vi "Jog_Home_Device_Travel_Range.vi"() -> ()   [LabVIEW 2017]
uses:
  U:/UDocuments/Thorlabs.Elliptec.ELLO_DLL.dll
  Thorlabs.Elliptec.ELLO_DLL.dll
panel:
  out "Stage Position (mm/degrees)":dbl
  out "?":string[](array[string])
  in  "Jog Step Size (mm/degrees)":dbl
  in  "Homing Direction":i32(ring)=48 items=["Linear, Clockwise"=48, "AntiClockwise"=49]
  in  "Device Address":string
  in  "?":bool
  in  "?":bool
  in  "Stop VI":bool
  in  "?":bool
  # "Notes:"
  # "This VI requires a linear or rotary stage. The homing direction is limited by the stage you are using. \nRotary stages can home clockwise or anticlockwise while linear stages must use the Linear, Clockwise option.\n\nIf, when running the VI for the first time, you get a popup as illustrated below, then click Browse and navigate to the \nThorlabs.Elliptec.ELLO_DLL.dll file in the ELLO software installation directory. This can be copied to the folder you are \nrunning the VI from."
  # "Thorlabs Hardware: ELL6, ELL9, ELL14, ELL17, ELL18, ELLB \nhttps://www.thorlabs.com/thorproduct.cfm?partnumber=ELL17\n\nDescription: This VI will enable you to control an Elliptec stage using the home and jog commands. It assumes that you know the device address of your stage. By default this will be 0 unless changed by a user. It can be any value in Hex from 0 to F. If the device address is unknown then this is most easily found through the ELLO software: \nhttps://www.thorlabs.com/software_pages/ViewSoftwarePage.cfm?Code=ELL"
  # "Instructions:"
  # "1) Connect your device to the USB Interface board via the ribbon cable. \n2) Connect power to the board and wait for approximately 10 seconds. As soon as the stage has power it will attempt a frequency search.\n     If the power is insufficient the board will not find the correct operating frequencies. This is why the USB is attached last.\n3) Connect the interface board to the PC via the USB cable.\n4) Open the VI, then enter the address of the device being used and select the homing direction you wish to use.\n5) Run the VI"
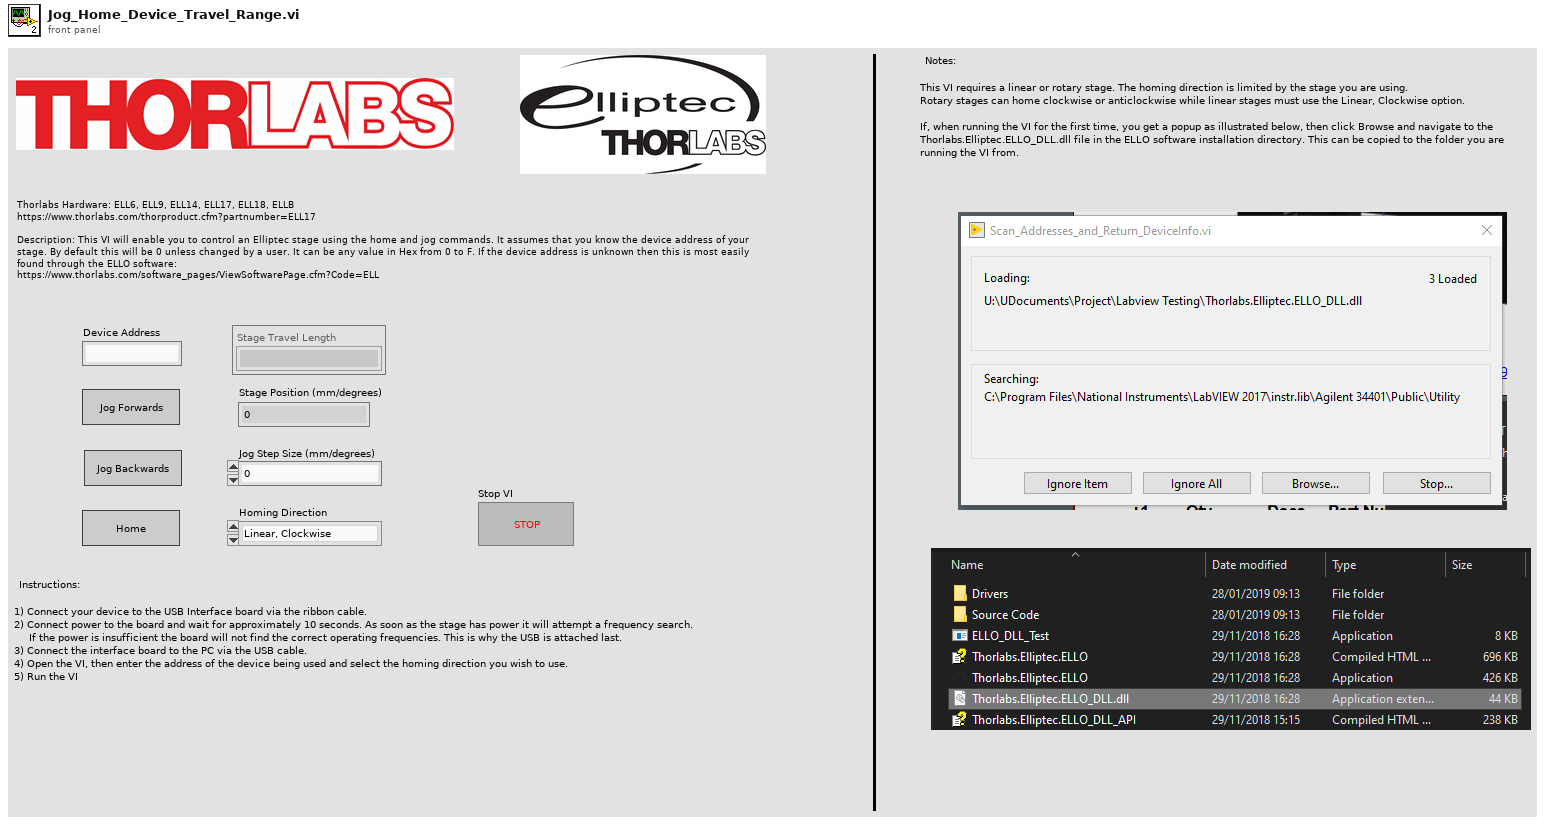
[diagram p1: front panel]
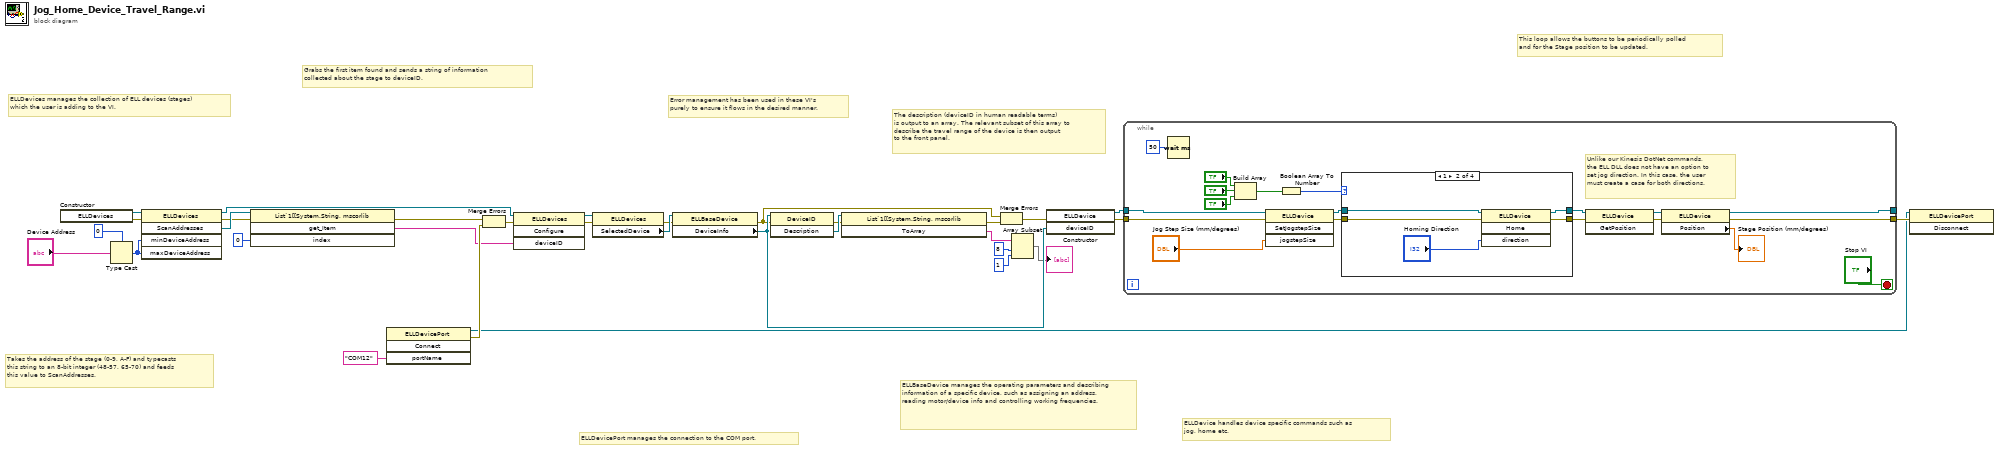
[diagram p0: block diagram]
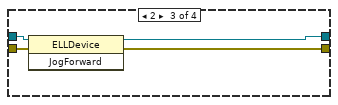
[diagram p3: hidden frame]
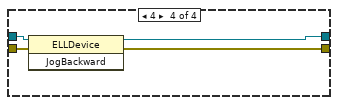
[diagram p4: hidden frame]
diagram:
  # "ELLBaseDevice manages the operating parameters and describing information of a specific device, such as assigning an address, reading motor/device info and controlling working frequencies."
  # "ELLDevice handles device specific commands such as \njog, home etc."
  # "Error management has been used in these VI's\npurely to ensure it flows in the desired manner."
  # "ELLDevices manages the collection of ELL devices (stages)\nwhich the user is adding to the VI."
  # "ELLDevicePort manages the connection to the COM port."
  # "This loop allows the buttons to be periodically polled \nand for the Stage position to be updated."
  # "The description (deviceID in human readable terms)\nis output to an array. The relevant subset of this array to\ndescribe the travel range of the device is then output \nto the front panel."
  # "Grabs the first item found and sends a string of information \ncollected about the stage to deviceID."
  # "Takes the address of the stage (0-9, A-F) and typecasts\nthis string to an 8-bit integer (48-57, 65-70) and feeds\nthis value to ScanAddresses."
  n1 = constructor class="ELLDevices"() -> (reference out=w21:refnum<k24>, error out=w13:errorcluster)  [unwired: 3 in, 1 out]
  n2 = Type Cast(type=u8 0 ("default (0 dbl)"), x="Device Address") -> (*(type *) &x=w19:u8)
  n3 = invoke class="ELLDevices" method="ScanAddresses"(reference=w21, error in=w13, "minDeviceAddress"=w19, "maxDeviceAddress"=w19) -> (reference out=w18:refnum<k24>, error out=w12:errorcluster, "ScanAddresses"=w15:refnum<k24>)  [unwired: 1 in, 2 out]
  n4 = invoke class="List`1[[System.String, mscorlib" method="get_Item"(reference=w15, error in=w12, "index"=0) -> (error out=w11:errorcluster, "get_Item"=w14:string)  [unwired: 1 in, 2 out]
  n5 = invoke class="ELLDevicePort" method="Connect"("portName"="COM12") -> (reference out=w22:refnum<k24>, error out=w29:errorcluster)  [unwired: 3 in, 2 out]
  n6 = Merge Errors(w11, w29) -> (w28:errorcluster)
  n7 = invoke class="ELLDevices" method="Configure"(reference=w18, error in=w28, "deviceID"=w14) -> (reference out=w31:refnum<k24>, error out=w27:errorcluster)  [unwired: 1 in, 2 out]
  n8 = property class="ELLDevices"(reference=w31, error in=w27) -> (error out=w26:errorcluster, "SelectedDevice"=w30:refnum<k24>)  [unwired: 1 out]
  n9 = property class="ELLBaseDevice"(reference=w30, error in=w26) -> (error out=w3:errorcluster, "DeviceInfo"=w10:refnum<k24>)  [unwired: 1 out]
  n10 = invoke class="DeviceID" method="Description"(reference=w10, error in=w3) -> (error out=w4:errorcluster, "Description"=w9:refnum<k24>)  [unwired: 1 in, 1 out]
  n11 = invoke class="List`1[[System.String, mscorlib" method="ToArray"(reference=w9, error in=w4) -> (error out=w2:errorcluster, "ToArray"=w1:string[])  [unwired: 1 in, 1 out]
  n12 = Merge Errors(w3, w2) -> (w5:errorcluster)
  n13 = Array Subset(array=w1, index=8, length=1) -> (→"?":string[])
  n14 = constructor class="ELLDevice"(error in=w5, "deviceID"=w10) -> (reference out=w25:refnum<k24>, error out=w24:errorcluster)  [unwired: 2 in, 2 out]
  n15 = while {
    tunnel: w25 -> [w42]
    tunnel: [w34] -> _
    tunnel: w24 -> [w41]
    tunnel: [w33] -> w23
    stop <- "Stop VI" stop-if-true
    # "Unlike our Kinesis DotNet commands,\nthe ELL DLL does not have an option to\nset jog direction. In this case, the user\nmust create a case for both directions."
    n16 = Wait (ms)(milliseconds to wait=u32 50) -> ()  [unwired: 1 out]
    n17 = Build Array("?", "?", "?") -> (w51:bool[])
    n18 = invoke class="ELLDevice" method="SetJogstepSize"(reference=w42, error in=w41, "jogstepSize"="Jog Step Size (mm/degrees)") -> (reference out=w43:refnum<k24>, error out=w40:errorcluster)  [unwired: 1 in, 2 out]
    n19 = Boolean Array To Number(Boolean array=w51) -> (number=w50:u32)
    n20 = case shown="1" w50 {
      tunnel: w43 -> [w53 w57 w62 w66]
      tunnel: [w53 w58 w61 w63] -> w36
      tunnel: w40 -> [w52 w56 w59 w65]
      tunnel: [w52 w55 w60 w64] -> w35
      frame 0, Default {
      }
      frame 1 {
        n21 = invoke class="ELLDevice" method="Home"(reference=w57, error in=w56, "direction"="Homing Direction") -> (reference out=w58:refnum<k24>, error out=w55:errorcluster)  [unwired: 1 in, 2 out]
      }
      frame 2 {
        n22 = invoke class="ELLDevice" method="JogForward"(reference=w62, error in=w59) -> (reference out=w61:refnum<k24>, error out=w60:errorcluster)  [unwired: 1 in, 1 out]
      }
      frame 4 {
        n23 = invoke class="ELLDevice" method="JogBackward"(reference=w66, error in=w65) -> (reference out=w63:refnum<k24>, error out=w64:errorcluster)  [unwired: 1 in, 1 out]
      }
    }
    n24 = invoke class="ELLDevice" method="GetPosition"(reference=w36, error in=w35) -> (reference out=w38:refnum<k24>, error out=w37:errorcluster)  [unwired: 1 in, 1 out]
    n25 = property class="ELLDevice"(reference=w38, error in=w37) -> (reference out=w34:refnum<k24>, error out=w33:errorcluster, "Position"=→"Stage Position (mm/degrees)":dbl)
  }
  n26 = invoke class="ELLDevicePort" method="Disconnect"(reference=w22, error in=w23) -> ()  [unwired: 1 in, 3 out]
